vi "Get Plugin Thread Interfaces.vi"(11 "Plugin Interface Pool in":refnum<class "Plugin Interface Pool.lvclass">) -> (2 "Plugin Thread Interfaces":refnum<class "Plugin Interface.lvclass">[](array[class]), 3 "Plugin Interface Pool out":refnum<class "Plugin Interface Pool.lvclass">)   [LabVIEW 2017, in "DSF Core.lvlib" / "Plugin Interface Pool.lvclass"]
uses:
  Plugin Interface Pool.lvclass
  Interfaces/Transceiver Interface/Plugin Interface.lvclass
  Plugin Interface Pool.lvclass/Plugin Interface Pool.ctl
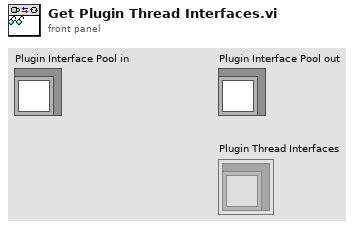
[diagram p1: front panel]
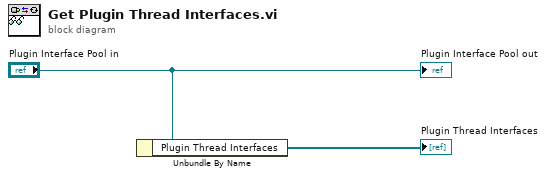
[diagram p0: block diagram]
diagram:
  n1 = Unbundle By Name("Plugin Interface Pool in") -> ("Plugin Thread Interfaces"=→"Plugin Thread Interfaces":refnum<class "Plugin Interface.lvclass">[])
  "Plugin Interface Pool out" <- "Plugin Interface Pool in"
